vi "get_config_cluster.vi"(8 "error in (no error)":errorcluster, 11 "GenericPlugin in":refnum<class "DisplayDL090216.lvclass">) -> (0 "error out":errorcluster, 2 "config cluster (variant)":variant, 3 "GenericPlugin out":refnum<class "DisplayDL090216.lvclass">)   [LabVIEW 2010, in "DisplayDL090216.lvclass"]
uses:
  DisplayDL090216.lvclass
  DisplayDL090216.lvclass/DisplayDL090216.ctl
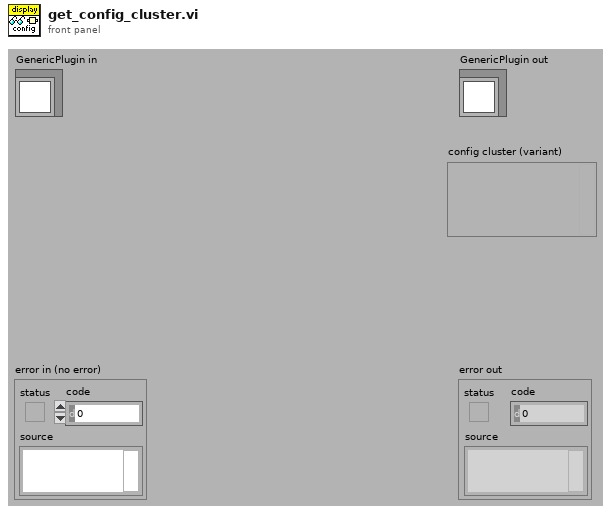
[diagram p1: front panel]
types:
  T1 = typedef "DisplayDL090216.lvclass/config_data_cluster.ctl" = cluster{"image processors":T2[], "range/offset processor configuration":string, "number of channels":i32, "autoscale cluster":cluster{"autoscale histogram":bool, "channel_1_min":dbl, "channel_1_max":dbl, "channel_2_min":dbl, "channel_2_max":dbl, "channel_3_min":dbl, "channel_3_max":dbl, "enable histogram?":bool}}
  T2 = typedef "plugin_specification.ctl" = cluster{"class path":string, "configuration":string, "label":string, "settings name":string}
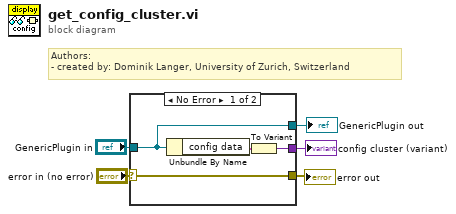
[diagram p0: block diagram]
diagram:
  # "Authors: \n- created by: Dominik Langer, University of Zurich, Switzerland"
  n1 = case shown="No Error" "error in (no error)" {
    selector: "error in (no error)" -> [w8 w11]
    tunnel: "GenericPlugin in" -> [w7 w10]
    tunnel: [w8 w11] -> w5
    tunnel: [w7 w10] -> w4
    tunnel: [w6 _] -> w1
    frame No Error {
      n2 = Unbundle By Name(w7) -> ("config data"=w9:T1)
      n3 = To Variant(anything=w9) -> (Variant=w6:variant)
    }
    frame Error {
    }
  }
  "error out" <- w5
  "GenericPlugin out" <- w4
  "config cluster (variant)" <- w1
